vi "temp.vi"() -> ()   [LabVIEW 2021]
uses:
  IMU Display.lvlib
  <vilib>/Platform/TimedLoop/XDataNode/wakeup.ctl
  <vilib>/Platform/TimedLoop/XDataNode/XDNodeRunTimeDep.lvlib
  <vilib>/Platform/TimedLoop/XDataNode/nitl_modes.ctl
  <vilib>/Platform/TimedLoop/XDataNode/timing_clust.ctl
  <vilib>/platform/TimedLoop/XDataNode/XDataNode.xnode
  <vilib>/picture/3D Picture Control/NI_3D Picture Control.lvlib
panel:
  out "Euler angles":dbl[](array[numeric])
  in  "y":i32=10
  out "Array":dbl[](array[numeric])
  in  "ZYX":bool
  in  "x":dbl[](array[numeric])
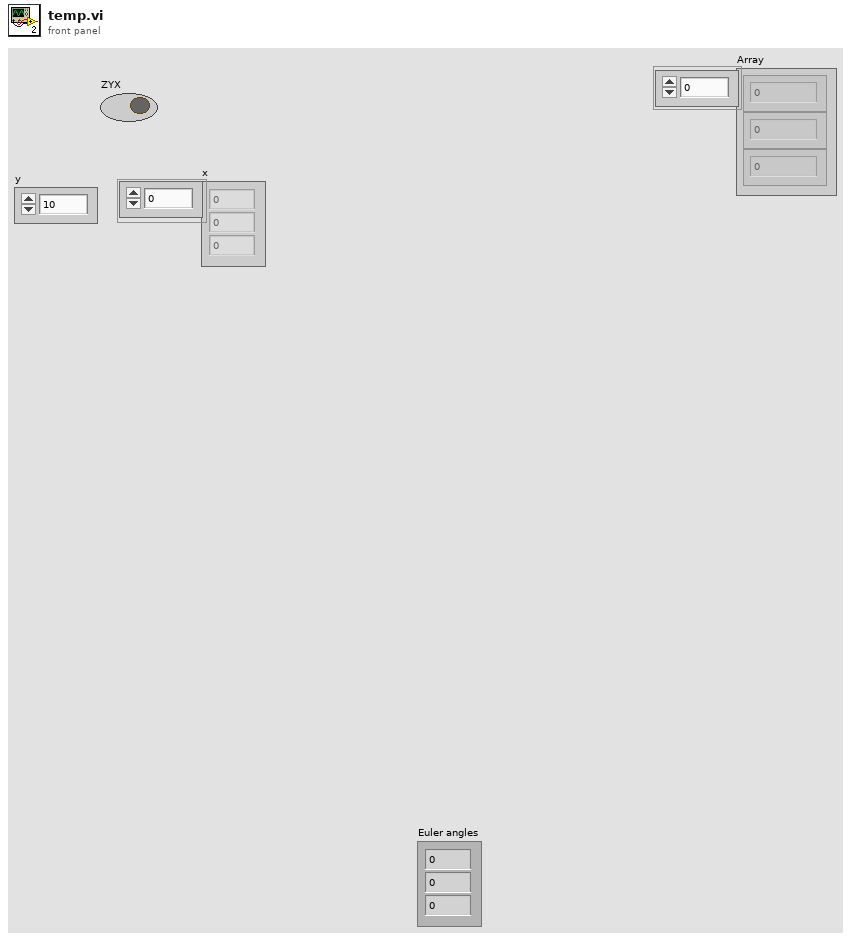
[diagram p1: front panel]
types:
  T1 = typedef "XDNodeRunTimeDep.lvlib/timing_clust.ctl" = cluster{"Expected End [f-1]":u64, "Actual End [f-1]":u64, "Finished Late? [f-1]":bool, "Expected End [i-1]":u64, "Actual End [i-1]":u64, "Finished Late? [i-1]":bool, "Expected Start [i]":u64, "Actual Start [i]":u64, "Expected Start [f]":u64, "Actual Start [f]":u64, "Source Name":string, "Structure Name":string, "Period":i64, "Deadline":i64, "Offset":i64, "Start":i64, "Priority":i32, "Timeout":i32, "Mode":T2, "Wakeup Reason":T3, "Error":errorcluster, "Source Type":string, "Secondary Source Type":string, "Global End Time":u64, "Global Start Time":u64, "Frame Duration":u64, "Iteration Duration":u64, "Assigned CPU":i32, "I/O Scan Engine Mode":u32}
  T2 = typedef "XDNodeRunTimeDep.lvlib/nitl_modes.ctl" = enum32{"No Change", "Process missed periods, maintain original phase", "Discard missed periods, maintain original phase", "Process missed periods, ignore original phase", "Discard missed periods, ignore original phase"}
  T3 = typedef "XDNodeRunTimeDep.lvlib/wakeup.ctl" = enum32{"Normal", "Aborted", "Asynchronous wakeup", "Timing source error", "Timed loop error", "Timeout"}
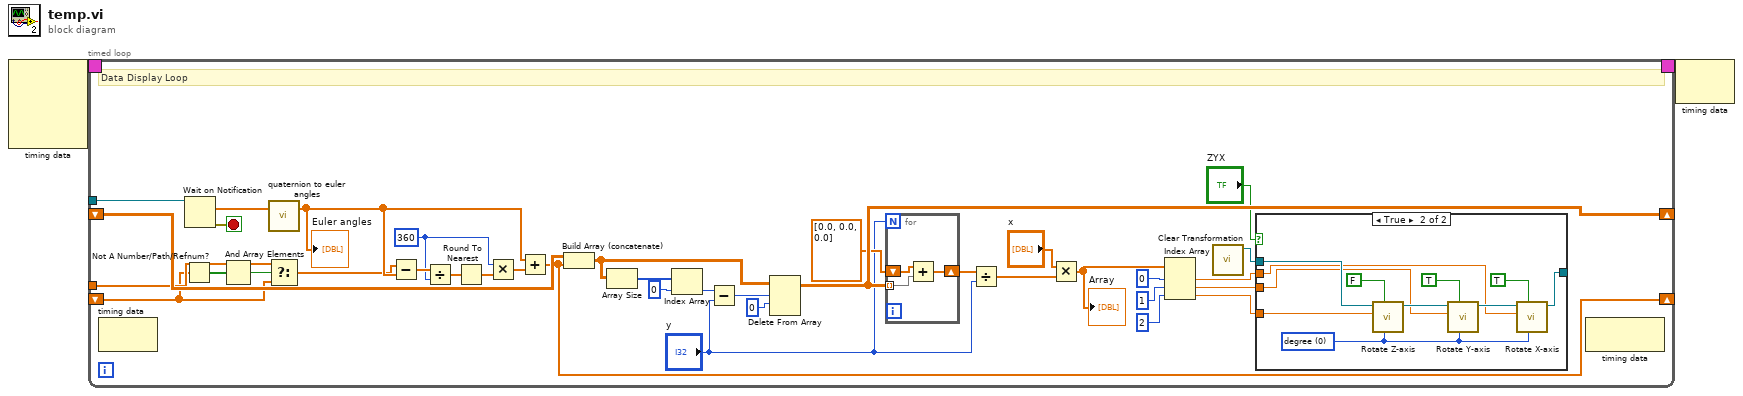
[diagram p0: block diagram]
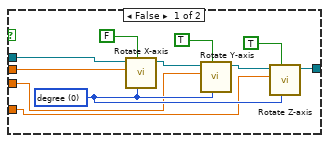
[diagram p2: hidden frame]
diagram:
  n1 = node-c288() -> (w2:T1)  [unwired: 4 in]
  n2 = timed-loop "Data Display Loop" {
    tunnel: _ -> [w39]
    timing: w2 -> [_]
    timing-out: [_] -> w1
    shift-right: [w26] -> _
    shift-left: _ -> [w15]
    shift-right: [w8] -> _
    shift-left: _ -> [w3]
    tunnel: _ -> [w4]
    stop <- w38 stop-if-true
    w9 = 360
    # "Data Display Loop"
    n3 = node-c288() -> ()  [unwired: 1 in, 1 out]
    n4 = Not A Number/Path/Refnum?(number/path/refnum=w3) -> (NaN/Path/Refnum?=w6:bool[])
    n5 = Wait on Notification(notifier=w39) -> (notification=w37:dbl[], error out=w38:errorcluster)  [unwired: 3 in, 2 out]
    n6 = And Array Elements(Boolean array=w6) -> (logical AND=w5:bool)
    n7 = call "quaternion to euler angles.vi"("Quaternion"=w37) -> ("Euler angles"=w12:dbl[])  [unwired: 2 in]
    "Euler angles" <- w12
    n8 = Select(t=w4, s=w5, f=w3) -> (s? t:f=w7:dbl[])
    n9 = Subtract(x=w7, y=w12) -> (x-y=w14:dbl[])
    n10 = Divide(x=w14, y=w9) -> (x/y=w13:dbl[])
    n11 = Round To Nearest(number=w13) -> (nearest integer value=w10:dbl[])
    n12 = Multiply(x=w9, y=w10) -> (x*y=w11:dbl[])
    n13 = Add(x=w12, y=w11) -> (x+y=w8:dbl[])
    n14 = Build Array (concatenate)(w15, w8) -> (w32:dbl[][])
    n15 = Array Size(array=w32) -> (size(s)=w31:i32[])
    n16 = Index Array(array=w31, index=0) -> (element=w29:i32)
    n17 = Subtract(x=w29, y="y") -> (x-y=w28:i32)
    n18 = Delete From Array(array=w32, length=w28, index (row)=0) -> (array with subset deleted=w26:dbl[][])  [unwired: 1 in, 1 out]
    n19 = for {
      N: "y" -> [_]
      tunnel: w26 -> [w64] mode=indexing
      shift-right: [w63] -> w24
      shift-left: dbl[] [0.0, 0.0, 0.0] -> [w62]
      n20 = Add(x=w62, y=w64) -> (x+y=w63:dbl[])
    }
    n21 = Divide(x=w24, y="y") -> (x/y=w22:dbl[])
    n22 = Multiply(x="x", y=w22) -> (x*y=w17:dbl[])
    "Array" <- w17
    n23 = Index Array(array=w17, index #1=0 ("index"), index #2=1 ("index"), index #3=2 ("index")) -> (element #1=w21:dbl, element #2=w20:dbl, element #3=w19:dbl)
    n24 = call <vilib>:"Clear Transformation.vi"() -> ("Object Refnum Out"=w36:refnum<vi>)  [unwired: 10 in, 1 out]
    n25 = case shown="True" "ZYX" {
      tunnel: [w40 w60] -> _
      tunnel: w36 -> [w41 w56]
      tunnel: w21 -> [w44 w53]
      tunnel: w20 -> [w43 w52]
      tunnel: w19 -> [w42 w51]
      frame False {
        w50 = u16 0 items=["degree", "radians"] ("angle unit")
        n26 = call <vilib>:"Rotate X-axis.vi"("angle unit"=w50, "Relative?"=FALSE, "angle"=w44, "Scene Object In"=w41) -> ("Scene Object Out"=w47:refnum<vi>)  [unwired: 6 in, 1 out]
        n27 = call <vilib>:"Rotate Y-axis.vi"("angle unit"=w50, "Relative?"=TRUE, "angle"=w43, "Scene Object In"=w47) -> ("Scene Object Out"=w49:refnum<vi>)  [unwired: 6 in, 1 out]
        n28 = call <vilib>:"Rotate Z-axis.vi"("angle unit"=w50, "Relative?"=TRUE, "angle"=w42, "Scene Object In"=w49) -> ("Scene Object Out"=w40:refnum<vi>)  [unwired: 6 in, 1 out]
      }
      frame True {
        w61 = u16 0 items=["degree", "radians"] ("angle unit")
        n29 = call <vilib>:"Rotate Z-axis.vi"("angle unit"=w61, "Relative?"=FALSE, "angle"=w51, "Scene Object In"=w56) -> ("Scene Object Out"=w57:refnum<vi>)  [unwired: 6 in, 1 out]
        n30 = call <vilib>:"Rotate Y-axis.vi"("angle unit"=w61, "Relative?"=TRUE, "angle"=w52, "Scene Object In"=w57) -> ("Scene Object Out"=w59:refnum<vi>)  [unwired: 6 in, 1 out]
        n31 = call <vilib>:"Rotate X-axis.vi"("angle unit"=w61, "Relative?"=TRUE, "angle"=w53, "Scene Object In"=w59) -> ("Scene Object Out"=w60:refnum<vi>)  [unwired: 6 in, 1 out]
      }
    }
    n32 = node-c288() -> ()  [unwired: 1 in, 1 out]
  }
  n33 = node-c288(w1) -> ()  [unwired: 1 out]
